vi "TurnAndZerov2.vi"   [LabVIEW 2015]
types:
  T1 = typedef "WPI_MotorControlDeviceRef.ctl" = cluster{"DeviceStatus":errorcluster, "Type":T2, "PWM":cluster{"PWM Channel":T3, "DeadBand":T4}, "CAN":cluster{"Device Number":u8, "Control Mode":T5, "Semaphore":T6, "Max Vout":dbl, "TalonSRX Control Mode":T7}, "Invert":bool}
  T2 = typedef "WPI_MotorControlType.ctl" = enum16{"PWM", "CAN", "CANTalonSRX"}
  T3 = typedef "FPGA_DIOPWMChannel.ctl" = enum8{"PWM 0", "PWM 1", "PWM 2", "PWM 3", "PWM 4", "PWM 5", "PWM 6", "PWM 7", "PWM 8", "PWM 9", "PWM MXP 0", "PWM MXP 1", "PWM MXP 2", "PWM MXP 3", "PWM MXP 4", "PWM MXP 5", "PWM MXP 6", "PWM MXP 7", "PWM MXP 8", "PWM MXP 9", "Invalid"}
  T4 = typedef "WPI_PWMDeadband.ctl" = cluster{"Name":string, "maxPositivePwm":i32, "minPositivePwm":i32, "centerPwm":i32, "maxNegativePwm":i32, "minNegativePwm":i32, "angularRange":u16}
  T5 = typedef "WPI_CANJaguar_ControlMode.ctl" = enum8{"Percent VBus", "Current", "Speed", "Position", "Voltage"}
  T6 = typedef "Semaphore RefNum" = refnum<k1>
  T7 = typedef "WPI_CANTalonSRX_APIControlMode.ctl" = enum8{"Percent VBus", "Speed", "Position", "Slave", "Unchanged / Invalid", "Voltage Compensation", "Current", "Motion Profile"}
  T8 = typedef "WPI_CANTalonSRX_GlobalStatus.ctl" = cluster{"Applied Throttle":dbl, "Module Enabled":bool, "CAN Error":errorcluster, "Closed Loop Error":dbl, "Forward Limit Switch Closed":bool, "Reverse Limit Switch Closed":bool, "Sensor Position":dbl, "Sensor Velocity":dbl, "Current":dbl, "Sticky Fault - Over Temp":bool, "Sticky Fault - Under Voltage":bool, "Sticky Fault - Forward Limit":bool, "Sticky Fault - Reverse Limit":bool, "Sticky Fault - Forward Soft Limit":bool, "Sticky Fault - Reverse Soft Limit":bool, "Brake is Enabled":bool, "Encoder Position":dbl, "Encoder Velocity":dbl, "Encoder Index Count":dbl, "Encoder A Pin State":bool, "Encoder B Pin State":bool, "Encoder Index Pin State":bool, "Analog In":dbl, "Analog In Velocity":dbl, "Temperature (C)":dbl, "Battery Voltage":dbl, "Control 5 Is Supported":bool, "Current Profile Slot Select":dbl, "Pos Div 8":bool, "Vel Div 4":bool, "Pulse Width Position":i32, "Pulse Width Velocity":i32, "Pulse Width Rise To Rise (us)":i32, "Pulse Width Rise To Fall (us)":i32, "Mot Prof Active Is Under Run":bool, "Mot Prof Active Has Under Run":bool, "Mot Prof Active Is Last":bool, "Mot Prof Active Velocity Only":bool, "Mot Prof Active Is Valid":bool, "Mot Prof Buffer Is Full":bool, "Mot Prof Active Profile Slot Select":i32, "Mot Prof NextID":i32, "Mot Prof Count":i32, "Mot Prof Active Velocity":dbl, "Mot Prof Active Position":dbl, "Mot Prof Output Enable":i32}
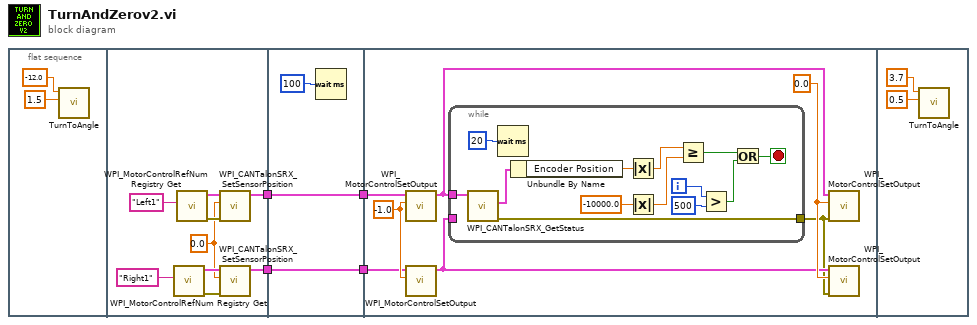
[diagram p0: block diagram]
diagram:
  n1 = flat-sequence {
    tunnel: [w8] -> w3
    tunnel: [w7] -> w1
    tunnel: [w17] -> w4
    tunnel: w3 -> [w17]
    tunnel: [w16] -> w2
    tunnel: w1 -> [w16]
    tunnel: w4 -> [w20]
    tunnel: w2 -> [w19]
    frame #0 {
      n2 = call "TurnToAngle.vi"("AllowedDeviation"=1.5, "GyroValue"=-12.0) -> ()  [unwired: 10 in]
    }
    frame #1 {
      w9 = 0.0 ("New Sensor Position")
      n3 = call <vilib>:"WPI_MotorControlRefNum Registry Get.vi"("refnum name"="Right1") -> ("error out"=w13:errorcluster, "MotorControlDevRef"=w12:T1)  [unwired: 9 in]
      n4 = call <vilib>:"WPI_MotorControlRefNum Registry Get.vi"("refnum name"="Left1") -> ("error out"=w11:errorcluster, "MotorControlDevRef"=w10:T1)  [unwired: 9 in]
      n5 = call <vilib>:"WPI_CANTalonSRX_SetSensorPosition.vi"("error in (no error)"=w11, "New Sensor Position"=w9, "CAN Talon SRX Ref"=w10) -> ("CAN Talon SRX Ref"=w7:T1)  [unwired: 7 in, 1 out]
      n6 = call <vilib>:"WPI_CANTalonSRX_SetSensorPosition.vi"("error in (no error)"=w13, "New Sensor Position"=w9, "CAN Talon SRX Ref"=w12) -> ("CAN Talon SRX Ref"=w8:T1)  [unwired: 7 in, 1 out]
    }
    frame #2 {
      n7 = Wait (ms)(milliseconds to wait=u32 100) -> ()  [unwired: 1 out]
    }
    frame #3 {
      w22 = -1.0 ("Output")
      w25 = 0.0 ("Output")
      n8 = call <vilib>:"WPI_MotorControlSetOutput.vi"("Output"=w22, "MotorControlDevRef"=w19) -> ("MotorControlDevRef"=w24:T1)  [unwired: 7 in, 2 out]
      n9 = call <vilib>:"WPI_MotorControlSetOutput.vi"("Output"=w22, "MotorControlDevRef"=w20) -> ("MotorControlDevRef"=w23:T1)  [unwired: 7 in, 2 out]
      n10 = while {
        tunnel: w23 -> [_]
        tunnel: w24 -> [w28]
        tunnel: [w26] -> w21
        i -> [w33]
        stop <- w35 stop-if-true
        n11 = call <vilib>:"WPI_CANTalonSRX_GetStatus.vi"("CAN Talon SRX Ref"=w28) -> ("error out"=w26:errorcluster, "Talon SRX Status"=w37:T8)  [unwired: 8 in, 1 out]
        n12 = Wait (ms)(milliseconds to wait=u32 20) -> ()  [unwired: 1 out]
        n13 = Unbundle By Name(w37) -> ("Encoder Position"=w31:dbl)
        n14 = Absolute Value(x=w31) -> (abs(x)=w30:dbl)
        n15 = Absolute Value(x=-10000.0) -> (abs(x)=w29:dbl)
        n16 = Greater Or Equal?(x=w30, y=w29) -> (x >= y?=w36:bool)
        n17 = Greater?(x=w33, y=500) -> (0:w34:bool)
        n18 = Or(x=w36, y=w34) -> (x .or. y?=w35:bool)
      }
      n19 = call <vilib>:"WPI_MotorControlSetOutput.vi"("error in (no error)"=w21, "Output"=w25, "MotorControlDevRef"=w24) -> ()  [unwired: 6 in, 3 out]
      n20 = call <vilib>:"WPI_MotorControlSetOutput.vi"("error in (no error)"=w21, "Output"=w25, "MotorControlDevRef"=w23) -> ()  [unwired: 6 in, 3 out]
    }
    frame #4 {
      n21 = call "TurnToAngle.vi"("AllowedDeviation"=0.5, "GyroValue"=3.7) -> ()  [unwired: 10 in]
    }
  }
